vi "Record Nested.vi"(8 "error in (no error)":errorcluster, 10 "Nested Queue":refnum<class "Priority Message Queue.lvclass">, 11 "Actor in":refnum<class "Actor.lvclass">) -> (0 "error out":errorcluster, 3 "Actor out":refnum<class "Actor.lvclass">)   [LabVIEW 2020, in "Artifex.lvlib" / "Actor.lvclass"]
uses:
  Actor.lvclass
  Actor Proxy/Actor API.lvclass
  Priority Message Queue/Priority Message Queue.lvclass
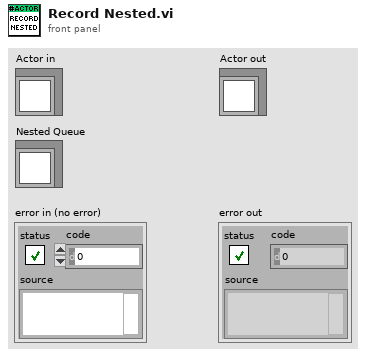
[diagram p1: front panel]
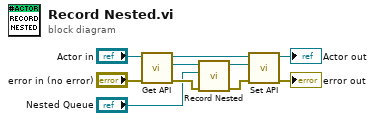
[diagram p0: block diagram]
diagram:
  n1 = call-dynamic "Get API.vi"("error in (no error)"="error in (no error)", "Actor in"="Actor in") -> ("error out"=w7:errorcluster, "Actor API"=w8:refnum<class "Actor API.lvclass">, "Actor out"=w5:refnum<class "Actor.lvclass">)  [unwired: 7 in]
  n2 = call "Record Nested.vi"("error in (no error)"=w7, "Nested Queue"="Nested Queue", "Actor API in"=w8) -> ("error out"=w3:errorcluster, "Actor API out"=w4:refnum<class "Actor API.lvclass">)  [unwired: 7 in]
  n3 = call-dynamic "Set API.vi"("error in (no error)"=w3, "Actor API"=w4, "Actor in"=w5) -> ("error out"=→"error out":errorcluster, "Actor out"=→"Actor out":refnum<class "Actor.lvclass">)  [unwired: 7 in]
